vi "PH_BL-Master.calc BL color.vi"(1 "State for \"2\" (on) of ABLE (off/false/out)":T1=1 items=["no info", "off/false/out", "on/true/in", "Failure", "Alarm", "Status 1", "Status 2", "Status 3"], 2 "State ABLE":T1 items=["no info", "off/false/out", "on/true/in", "Failure", "Alarm", "Status 1", "Status 2", "Status 3"], 3 "State before ABLE":i32) -> (0 "State after ABLE":i32)   [LabVIEW 2014, in "PH_BL-Master.lvlib"]
doc: "This VI is forseen to calculate the color of the actual beamline element (ABLE) behind shutters ect. This is of course depending on how the beamline before is looking like:\n\nIf the \"State before ABLE\" is 0, 1 or 6, the \"State after ABLE\" is the same.\n \nIf the \"State before ABLE\" is not 0, 1 or 6, and \"state ABLE\" is 1 or 2, the \"State after ABLE\" is \n= 1 if \"State ABLE\" equals \"State for \"2\" of ABLE\"\n= \"State before ABLE\" if \"State ABLE\" is not equal \"State for \"2\" of ABLE\"\n\nIf the \"State before ABLE\" is not 0, 1, or 6,, and \"state ABLE\" is not 1 or 2, the \"State after ABLE\" is 3."
uses:
  PH_BL-Master.lvlib
  PH_StatusHandler/PH_StatusHandler.Status.ctl
  PH_StatusHandler/PH_StatusHandler.lvlib
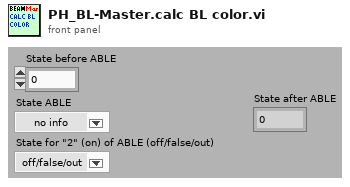
[diagram p1: front panel]
types:
  T1 = typedef "PH_StatusHandler.lvlib/PH_StatusHandler.Status.ctl" = i16
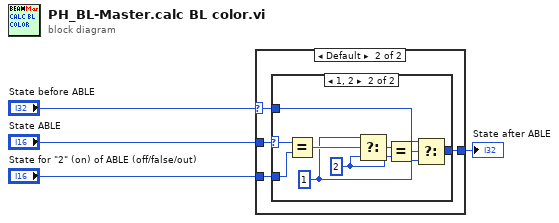
[diagram p0: block diagram]
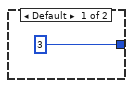
[diagram p3: hidden frame]
diagram:
  n1 = case shown="Default" "State before ABLE" {
    selector: "State before ABLE" -> [w5 w6]
    tunnel: [w5 w8] -> w2
    tunnel: "State for \"2\" (on) of ABLE (off/false/out)" -> [_ w9]
    tunnel: "State ABLE" -> [_ w7]
    frame 0, 1, 6 {
    }
    frame Default {
      n2 = case shown="1, 2" w7 {
        selector: w7 -> [_ w17]
        tunnel: w9 -> [_ w18]
        tunnel: [3 ("f") w13] -> w8
        tunnel: w6 -> [_ w16]
        frame Default {
        }
        frame 1, 2 {
          w11 = 1 ("f")
          w12 = 2 ("y")
          n3 = Equal?(x=w17, y=w18) -> (x = y?=w19:bool)
          n4 = Select(t=w11, s=w19, f=w12) -> (s? t:f=w14:i32)
          n5 = Equal?(x=w14, y=w12) -> (x = y?=w15:bool)
          n6 = Select(t=w16, s=w15, f=w11) -> (s? t:f=w13:i32)
        }
      }
    }
  }
  "State after ABLE" <- w2
